vi "Init.vi"(8 "error in (no error)":errorcluster, 10 "Node":refnum<class "Node.lvclass">) -> (0 "error out":errorcluster, 3 "Vecto out":refnum<class "Vecto.lvclass">)   [LabVIEW 2020, in "Vecto.lvlib" / "Vecto.lvclass"]
uses:
  Vecto.lvclass
  Node/Node.lvclass
  Vecto.lvclass/Vecto.ctl
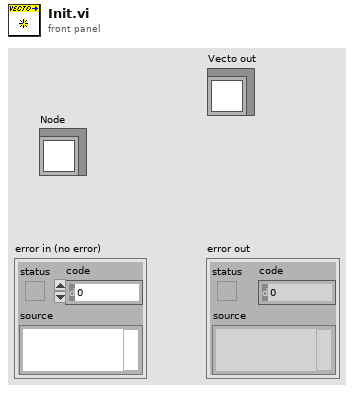
[diagram p1: front panel]
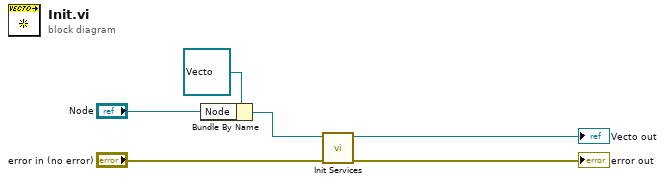
[diagram p0: block diagram]
diagram:
  n1 = Bundle By Name(cluster=refnum<class "Vecto.lvclass"> refnum ("Vecto in"), "Node"="Node") -> (w2:refnum<class "Vecto.lvclass">)
  n2 = call "Init Services.vi"("error in (no error)"="error in (no error)", "Vecto in"=w2) -> ("error out"=→"error out":errorcluster, "Vecto out"=→"Vecto out":refnum<class "Vecto.lvclass">)  [unwired: 8 in]
